vi "Probability calculation.vi"(1 "effective degrees of freedom":dbl, 2 "MSE array":dbl[](array[numeric]), 3 "Volumes":sgl[](array[numeric])) -> (0 "Sorted Probabilities":cluster{dbl, dbl, i32}[](array[cluster]))   [LabVIEW 2018]
panel:
  out "Array":dbl[](array[numeric])
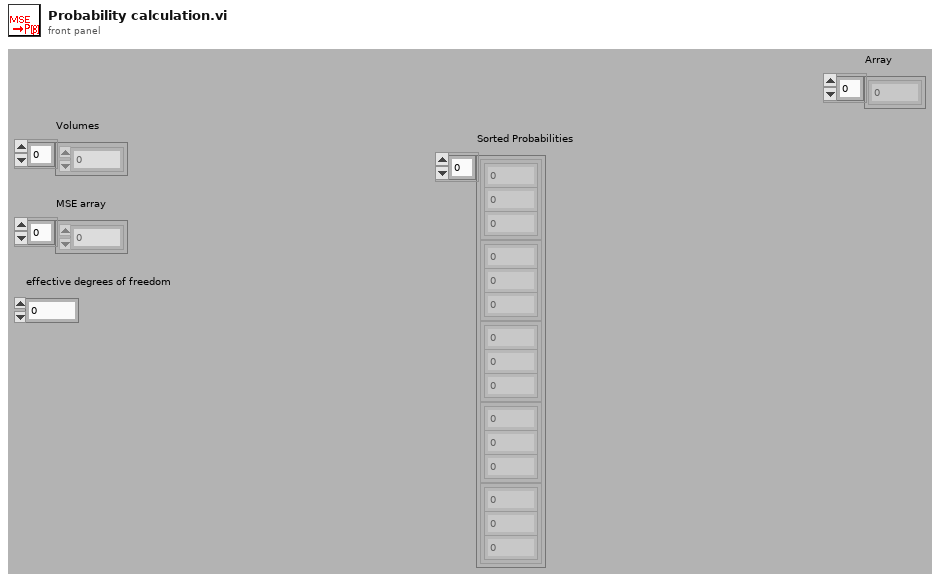
[diagram p1: front panel]
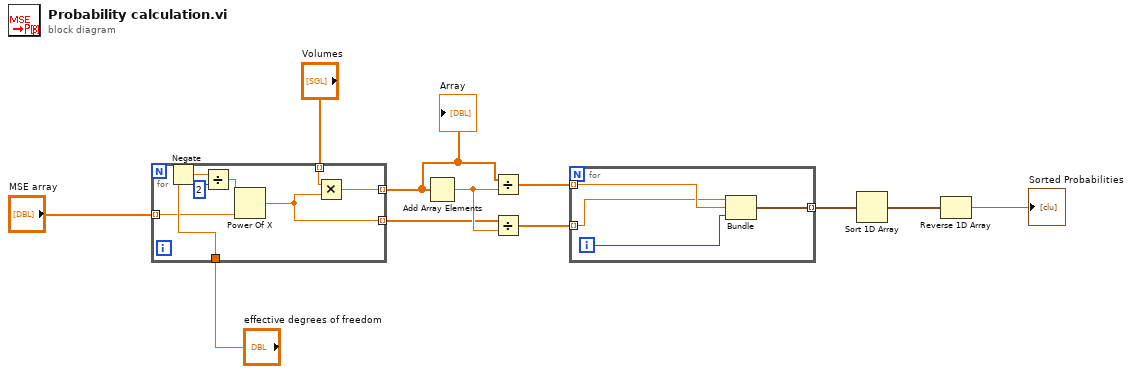
[diagram p0: block diagram]
diagram:
  n1 = for {
    tunnel: "MSE array" -> [w16] mode=indexing
    tunnel: [w14] -> w2 mode=indexing
    tunnel: "effective degrees of freedom" -> [w17]
    tunnel: "Volumes" -> [w13] mode=indexing
    tunnel: [w12] -> w9 mode=indexing
    n2 = Negate(x=w17) -> (-x=w19:dbl)
    n3 = Divide(x=w19, y=2 ("index")) -> (x/y=w15:dbl)
    n4 = Power Of X(1:w16, 2:w15) -> (0:w14:dbl)
    n5 = Multiply(x=w13, y=w14) -> (x*y=w12:dbl)
  }
  "Array" <- w9
  n6 = Add Array Elements(numeric array=w9) -> (sum=w8:dbl)
  n7 = Divide(x=w9, y=w8) -> (x/y=w7:dbl[])
  n8 = Divide(x=w2, y=w8) -> (x/y=w6:dbl[])
  n9 = for {
    tunnel: w7 -> [w23] mode=indexing
    tunnel: w6 -> [w20] mode=indexing
    tunnel: [w21] -> w5 mode=indexing
    i -> [w22]
    n10 = Bundle(w20, w23, w22) -> (w21:cluster{dbl, dbl, i32})  [unwired: 1 in]
  }
  n11 = Sort 1D Array(array=w5) -> (sorted array=w4:cluster{dbl, dbl, i32}[])
  n12 = Reverse 1D Array(array=w4) -> (reversed array=→"Sorted Probabilities":cluster{dbl, dbl, i32}[])
